vi "FM_Demodulation.vi"(8 "error in (no error)":errorcluster, 10 "Sample Rate (Hz)":u32=50000000 min=50000000 max=1800000000, 11 "Baseband Channel":T1) -> (0 "error out":errorcluster, 3 "Audio Channel Out":T2)   [LabVIEW 2016]
uses:
  <extravilib>/ChannelInstances/Stream-wfm(dbl)/)Channel.ctl
  <extravilib>/ChannelInstances/High Speed Stream-a[.](u8)/)Channel.ctl
  <vilib>/Analysis/3filter.llb/Filter Passband Type.ctl
  <extravilib>/ChannelInstances/High Speed Stream-a[.](u8)/_Read For Replicate.vi
  <extravilib>/ChannelInstances/Stream-wfm(dbl)/Write With Abort.vi
  <extravilib>/ChannelInstances/Stream-wfm(dbl)/Endpoint.vi
  <extravilib>/ChannelInstances/High Speed Stream-a[.](u8)/)Channel.vi
  <extravilib>/ChannelInstances/High Speed Stream-a[.](u8)/Abort Signal/Init Signal.vi
  <vilib>/Analysis/3filter.llb/Butterworth Filter (DBL).vi
  <vilib>/Analysis/2dsp.llb/Decimate (continuous, DBL).vi
  <extravilib>/ChannelInstances/Stream-wfm(dbl)/)Channel.vi
  <resource>/ChannelSupport/_ChannelSupport/WaitIfNeeded.vi
  <vilib>/Analysis/NI_AALBase.lvlib
  <extravilib>/ChannelInstances/Stream-wfm(dbl).lvlib
  <vilib>/Analysis/NI_AALPro.lvlib
  <extravilib>/ChannelInstances/High Speed Stream-a[.](u8).lvlib
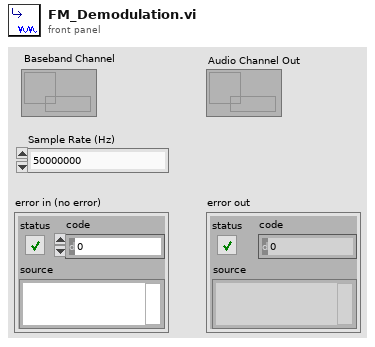
[diagram p1: front panel]
types:
  T1 = typedef "High Speed Stream-a[.](u8).lvlib/)Channel.ctl" = refnum<queue>
  T2 = typedef "Stream-wfm(dbl).lvlib/)Channel.ctl" = refnum<queue>
  T3 = typedef "NI_AALBase.lvlib/Filter Passband Type.ctl" = enum32{"Lowpass", "Highpass", "Bandpass", "Bandstop"}
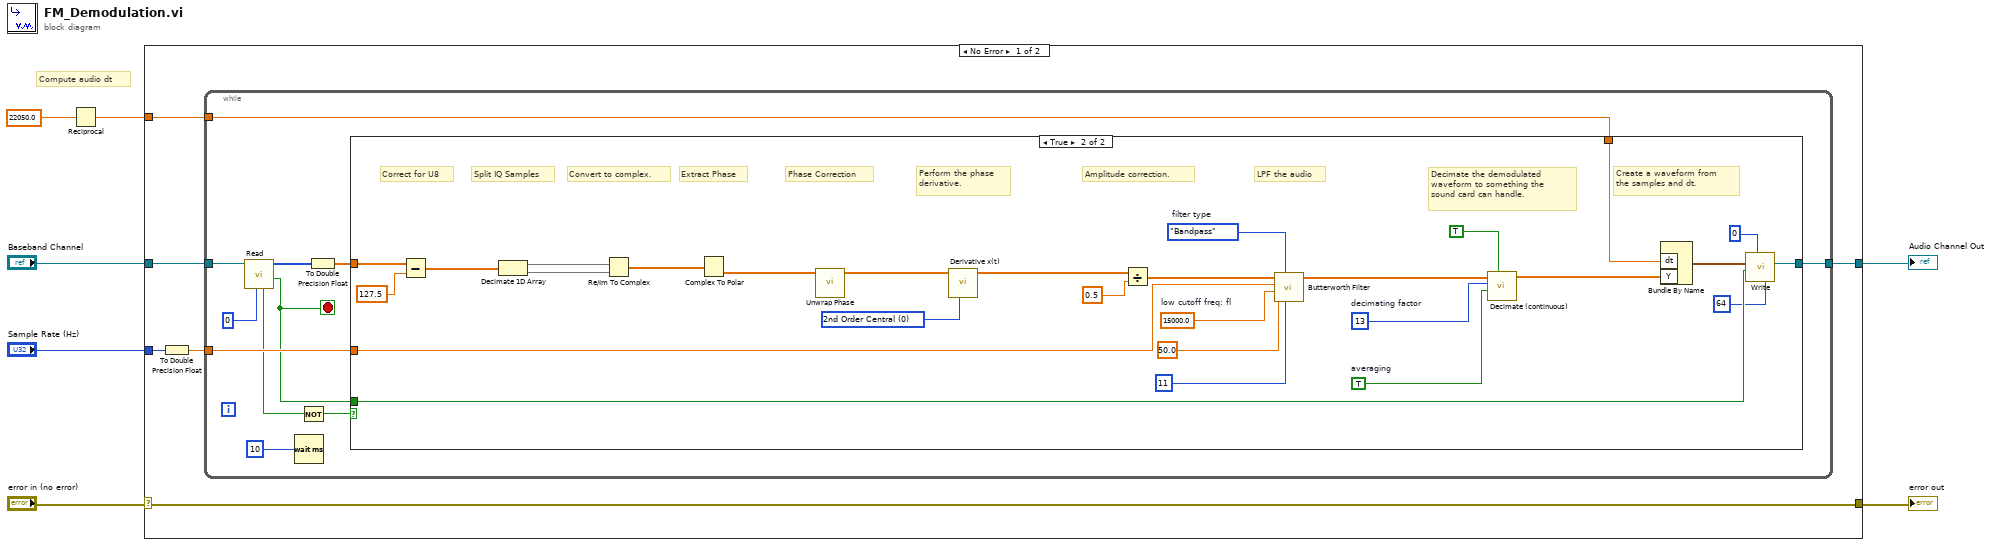
[diagram p0: block diagram]
diagram:
  # "Compute audio dt"
  n1 = Reciprocal(x=22050.0) -> (1/x=w6:dbl)
  n2 = case shown="No Error" "error in (no error)" {
    selector: "error in (no error)" -> [w10 w53]
    tunnel: "Sample Rate (Hz)" -> [w13 _]
    tunnel: w6 -> [w12 _]
    tunnel: [w10 w53] -> w3
    tunnel: [w9 _] -> w2
    tunnel: "Baseband Channel" -> [w8 _]
    frame No Error {
      n3 = To Double Precision Float(number=w13) -> (double precision float=w11:dbl)
      n4 = while {
        tunnel: [w24] -> w9
        tunnel: w11 -> [w22]
        tunnel: w12 -> [w20]
        tunnel: w8 -> [w15]
        stop <- w18 stop-if-true
        n5 = call <extravilib>:"Read.vi"("timeout in ms (-1)"=0, "channel"=w15) -> ("done?"=w18:bool, "element"=w17:u8[], "timed out?"=w14:bool)  [unwired: 5 in, 2 out]
        n6 = Wait (ms)(milliseconds to wait=u32 10) -> ()  [unwired: 1 out]
        n7 = Not(x=w14) -> (.not. x?=w19:bool)
        n8 = To Double Precision Float(number=w17) -> (double precision float=w23:dbl[])
        n9 = case shown="True" w19 {
          tunnel: [_ w50] -> w24
          tunnel: w23 -> [_ w49]
          tunnel: w22 -> [_ w29]
          tunnel: w20 -> [_ w44]
          tunnel: w18 -> [_ w35]
          frame False {
          }
          frame True {
            w34 = u16 0 items=["2nd Order Central", "4th Order Central", "Forward", "Backward"] ("method")
            w43 = TRUE  # averaging
            w42 = 13  # decimating factor
            w47 = Filter_Passband_Type."Bandpass"  # filter type
            w33 = 15000.0  # low cutoff freq: fl
            # "Decimate the demodulated\nwaveform to something the\nsound card can handle."
            # "Perform the phase\nderivative."
            # "Phase Correction"
            # "LPF the audio"
            # "Amplitude correction."
            # "Create a waveform from \nthe samples and dt."
            # "Correct for U8"
            # "Extract Phase"
            # "Convert to complex."
            # "Split IQ Samples"
            n10 = Subtract(x=w49, y=127.5) -> (x-y=w30:dbl[])
            n11 = Decimate 1D Array(w30) -> (w32:dbl[], w31:dbl[])
            n12 = Re/Im To Complex(1:w31, 2:w32) -> (0:w28:cdb[])
            n13 = Complex To Polar(r * e^(i*theta)=w28) -> (theta=w27:dbl[])  [unwired: 1 out]
            n14 = call <vilib>:"Unwrap Phase.vi"("Phase"=w27) -> ("Unwrapped Phase"=w38:dbl[])  [unwired: 9 in, 1 out]
            n15 = call <vilib>:"Derivative x(t).vi"("method"=w34, "X"=w38) -> ("dX/dt"=w37:dbl[])  [unwired: 8 in, 1 out]
            n16 = Divide(x=w37, y=0.5 ("dx/dt")) -> (x/y=w45:dbl[])
            n17 = call-poly <vilib>:"Butterworth Filter.vi"("order"=11, "filter type"=w47, "low cutoff freq: fl"=50.0, "high cutoff freq: fh"=w33, "sampling freq: fs"=w29, "X"=w45) -> ("Filtered X"=w40:dbl[])  [unwired: 2 in, 1 out]
            n18 = call-poly <vilib>:"Decimate (continuous).vi"("reset"=TRUE, "averaging"=w43, "decimating factor"=w42, "X"=w40) -> ("Decimated Array"=w39:dbl[])  [unwired: 6 in, 1 out]
            n19 = Bundle By Name("dt"=w44, "Y"=w39) -> (w36:waveform(dbl))  [unwired: 1 in]
            n20 = call <extravilib>:"Write.vi"("size (unlimited)"=64, "timeout in ms (-1)"=0, "last element? (F)"=w35, "element"=w36) -> ("channel"=w50:T2)  [unwired: 5 in, 2 out]
          }
        }
      }
    }
    frame Error {
    }
  }
  "error out" <- w3
  "Audio Channel Out" <- w2
